vi "SCM2_T_Control_Remote.vi"() -> ()   [LabVIEW 2018]
panel:
  out "Label.Text Array":string[](array[string])
  in  "Sorb Setpoint (K)":dbl=0.3 format="%#_4g"
  in  "OK Button":bool
  in  "Data mac ip address":string="146.201.200.173"
  in  "port":u16=3376
  in  "error in (no error) 2":errorcluster
  in  "Probe Setpoint (K)":dbl=0.3 format="%#_4g"
  in  "ico":u16(ring)=1 items=["Sorb"=1, "Probe"=2, "Test"=3]
  # "ico = 1 Sorb\n       = 2 Probe"
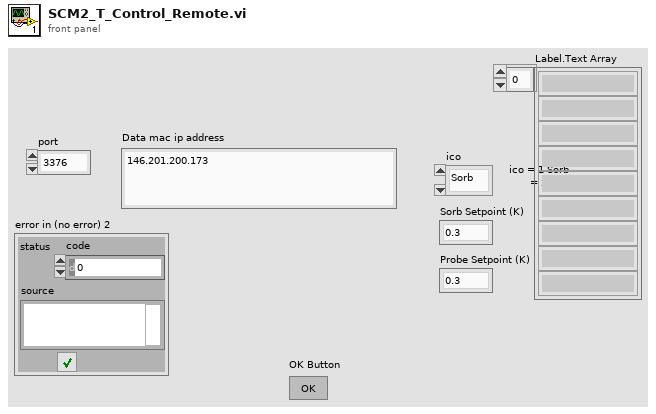
[diagram p1: front panel]
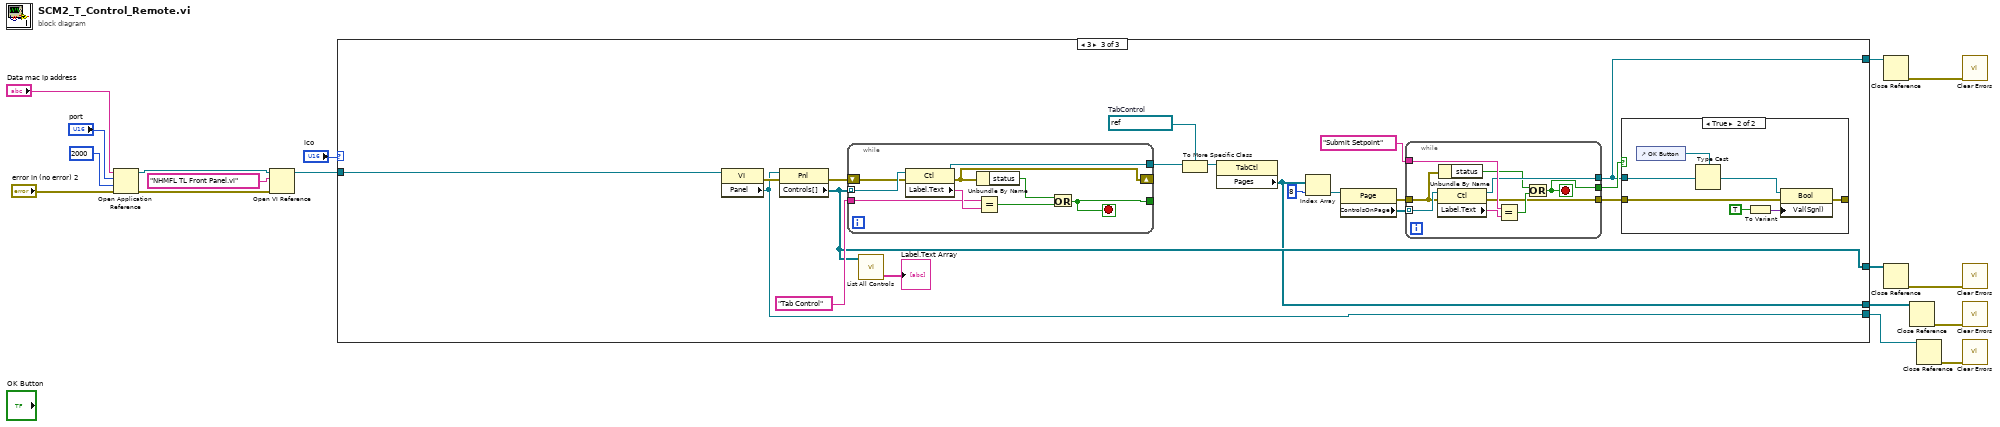
[diagram p0: block diagram]
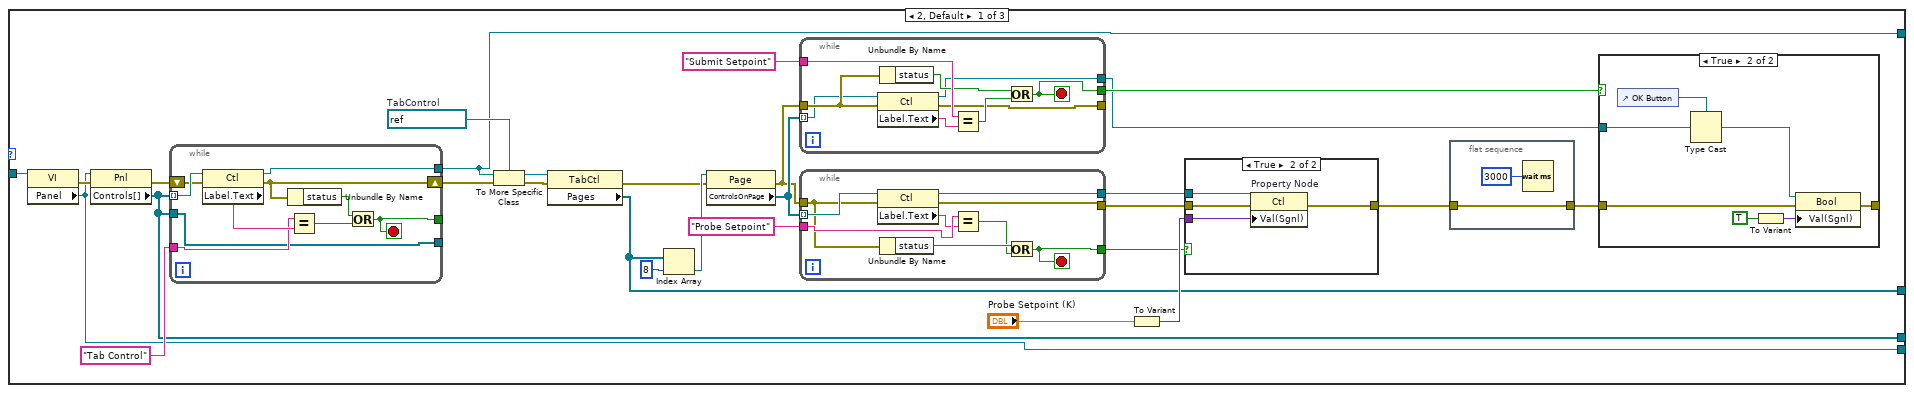
[diagram p2: hidden frame]
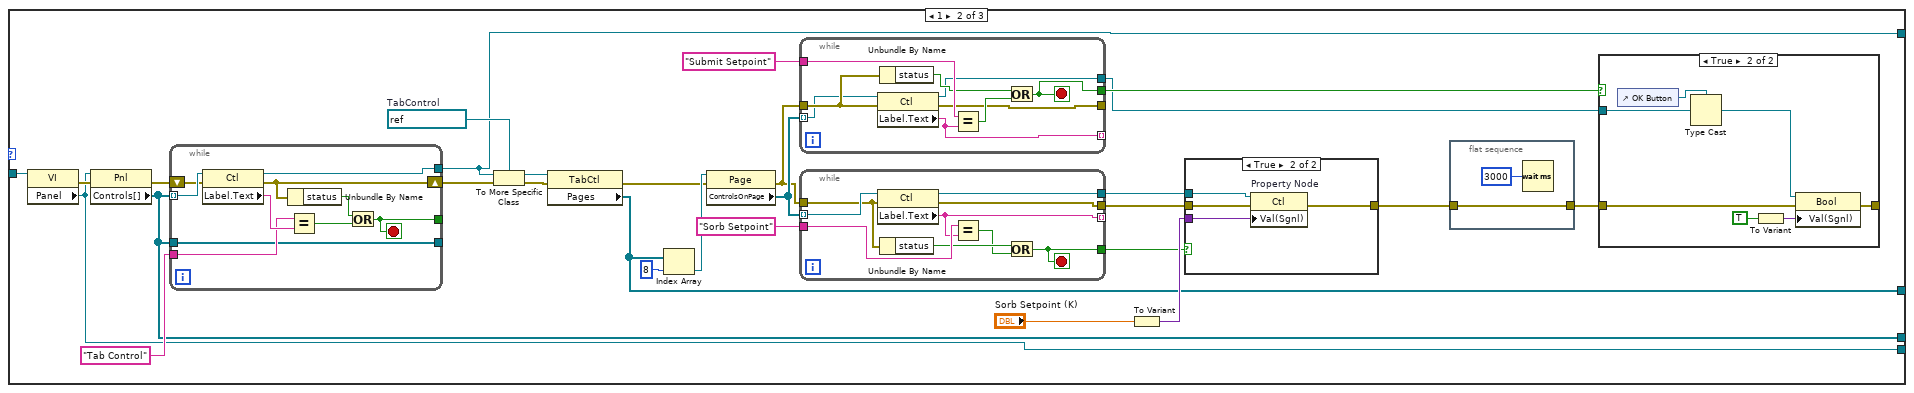
[diagram p5: hidden frame]
diagram:
  n1 = Open Application Reference(8:"error in (no error) 2", 9:2000 ("timeout ms (60000)"), 10:"port", 11:"Data mac ip address") -> (0:w4:errorcluster, 3:w5:refnum<vi>)
  n2 = Open VI Reference(application reference (local)=w5, vi path="NHMFL TL Front Panel.vi", error in (no error)=w4) -> (vi reference=w16:refnum<vi>)  [unwired: 3 in, 1 out]
  n3 = case shown="3" "ico" {
    tunnel: w16 -> [w41 w112 w177]
    tunnel: [w25 w94 w172] -> w13
    tunnel: [w26 w95 w160] -> w12
    tunnel: [w40 w111 w176] -> w11
    tunnel: [w24 w93 w161] -> w1
    frame 2, Default {
      w37 = refnum<vi> refnum  # TabControl
      n4 = property class="VI"(reference=w41) -> (error out=w45:errorcluster, "Panel"=w40:refnum<vi>)  [unwired: 1 in, 1 out]
      n5 = property class="Pnl"(reference=w40, error in=w45) -> (error out=w39:errorcluster, "Controls[]"=w26:refnum<vi>[])  [unwired: 1 out]
      n6 = while {
        tunnel: w26 -> [w88] mode=indexing
        tunnel: "Tab Control" ("Control Name") -> [w86]
        shift-right: [w83] -> w35
        shift-left: w39 -> [w85]
        tunnel: [w84] -> w25
        tunnel: [w80] -> _
        tunnel: w26 -> [w79]
        tunnel: [w79] -> _
        stop <- w80 stop-if-true
        n7 = property class="Ctl"(reference=w88, error in=w85) -> (reference out=w84:refnum<vi>, error out=w83:errorcluster, "Label.Text"=w87:string)
        n8 = Unbundle By Name(w83) -> ("status"=w82:bool)
        n9 = Equal?(x=w86, y=w87) -> (x = y?=w81:bool)
        n10 = Or(x=w82, y=w81) -> (x .or. y?=w80:bool)
      }
      n11 = To More Specific Class(target class=w37, reference=w25, error in=w35) -> (specific class reference=w38:refnum<vi>, error out=w36:errorcluster)
      n12 = property class="TabCtl"(reference=w38, error in=w36) -> (error out=w33:errorcluster, "Pages"=w24:refnum<vi>[])  [unwired: 1 out]
      n13 = Index Array(array=w24, index=8) -> (element=w34:refnum<vi>)
      n14 = property class="Page"(reference=w34, error in=w33) -> (error out=w18:errorcluster, "ControlsOnPage"=w19:refnum<vi>[])  [unwired: 1 out]
      n15 = while {
        tunnel: "Submit Setpoint" ("Control Name") -> [w56]
        tunnel: w18 -> [w51]
        tunnel: w19 -> [w49] mode=indexing
        tunnel: [w48] -> w22
        tunnel: [w53] -> w23
        tunnel: [w52] -> _
        stop <- w53 stop-if-true
        n16 = property class="Ctl"(reference=w49, error in=w51) -> (reference out=w48:refnum<vi>, error out=w52:errorcluster, "Label.Text"=w50:string)
        n17 = Unbundle By Name(w51) -> ("status"=w55:bool)
        n18 = Equal?(x=w56, y=w50) -> (x = y?=w54:bool)
        n19 = Or(x=w55, y=w54) -> (x .or. y?=w53:bool)
      }
      n20 = while {
        tunnel: "Probe Setpoint" ("Control Name") -> [w65]
        tunnel: w18 -> [w58]
        tunnel: w19 -> [w62] mode=indexing
        tunnel: [w61] -> w28
        tunnel: [w60] -> w30
        tunnel: [w59] -> w29
        stop <- w60 stop-if-true
        n21 = property class="Ctl"(reference=w62, error in=w58) -> (reference out=w61:refnum<vi>, error out=w59:errorcluster, "Label.Text"=w57:string)
        n22 = Unbundle By Name(w58) -> ("status"=w64:bool)
        n23 = Equal?(x=w65, y=w57) -> (x = y?=w63:bool)
        n24 = Or(x=w64, y=w63) -> (x .or. y?=w60:bool)
      }
      n25 = To Variant(anything="Probe Setpoint (K)") -> (Variant=w43:variant)
      n26 = case shown="True" w30 {
        tunnel: w29 -> [w74 w78]
        tunnel: [w74 w77] -> w21
        tunnel: w43 -> [_ w76]
        tunnel: w28 -> [_ w75]
        frame False {
        }
        frame True {
          n27 = property on="Property Node" class="Ctl"(reference=w75, error in=w78, "Val(Sgnl)"=w76) -> (error out=w77:errorcluster)  [unwired: 1 out]
        }
      }
      n28 = flat-sequence {
        tunnel: [w46] -> w20
        tunnel: w21 -> [w46]
        frame #0 {
          n29 = Wait (ms)(milliseconds to wait=u32 3000) -> ()  [unwired: 1 out]
        }
      }
      n30 = case shown="True" w23 {
        tunnel: w20 -> [w66 w72]
        tunnel: [w66 w71] -> _
        tunnel: w22 -> [_ w70]
        frame False {
        }
        frame True {
          n31 = control-ref of="OK Button"() -> (w73:refnum<vi>)
          n32 = Type Cast(type=w73, x=w70) -> (*(type *) &x=w69:refnum<vi>)
          n33 = To Variant(anything=TRUE) -> (Variant=w67:variant)
          n34 = property class="Bool"(reference=w69, error in=w72, "Val(Sgnl)"=w67) -> (error out=w71:errorcluster)  [unwired: 1 out]
        }
      }
    }
    frame 1 {
      w108 = refnum<vi> refnum  # TabControl
      n35 = property class="VI"(reference=w112) -> (error out=w116:errorcluster, "Panel"=w111:refnum<vi>)  [unwired: 1 in, 1 out]
      n36 = property class="Pnl"(reference=w111, error in=w116) -> (error out=w110:errorcluster, "Controls[]"=w95:refnum<vi>[])  [unwired: 1 out]
      n37 = while {
        tunnel: w95 -> [w159] mode=indexing
        tunnel: "Tab Control" ("Control Name") -> [w157]
        shift-right: [w154] -> w106
        shift-left: w110 -> [w156]
        tunnel: [w155] -> w94
        tunnel: [w151] -> _
        tunnel: w95 -> [w150]
        tunnel: [w150] -> _
        stop <- w151 stop-if-true
        n38 = property class="Ctl"(reference=w159, error in=w156) -> (reference out=w155:refnum<vi>, error out=w154:errorcluster, "Label.Text"=w158:string)
        n39 = Unbundle By Name(w154) -> ("status"=w153:bool)
        n40 = Equal?(x=w157, y=w158) -> (x = y?=w152:bool)
        n41 = Or(x=w153, y=w152) -> (x .or. y?=w151:bool)
      }
      n42 = To More Specific Class(target class=w108, reference=w94, error in=w106) -> (specific class reference=w109:refnum<vi>, error out=w107:errorcluster)
      n43 = property class="TabCtl"(reference=w109, error in=w107) -> (error out=w104:errorcluster, "Pages"=w93:refnum<vi>[])  [unwired: 1 out]
      n44 = Index Array(array=w93, index=8) -> (element=w105:refnum<vi>)
      n45 = property class="Page"(reference=w105, error in=w104) -> (error out=w97:errorcluster, "ControlsOnPage"=w98:refnum<vi>[])  [unwired: 1 out]
      n46 = while {
        tunnel: "Submit Setpoint" ("Control Name") -> [w127]
        tunnel: w97 -> [w122]
        tunnel: w98 -> [w120] mode=indexing
        tunnel: [w119] -> w91
        tunnel: [w124] -> w92
        tunnel: [w123] -> _
        tunnel: [w121] -> _ mode=indexing
        stop <- w124 stop-if-true
        n47 = property class="Ctl"(reference=w120, error in=w122) -> (reference out=w119:refnum<vi>, error out=w123:errorcluster, "Label.Text"=w121:string)
        n48 = Unbundle By Name(w122) -> ("status"=w126:bool)
        n49 = Equal?(x=w127, y=w121) -> (x = y?=w125:bool)
        n50 = Or(x=w126, y=w125) -> (x .or. y?=w124:bool)
      }
      n51 = while {
        tunnel: "Sorb Setpoint" ("Control Name") -> [w136]
        tunnel: w97 -> [w129]
        tunnel: w98 -> [w133] mode=indexing
        tunnel: [w132] -> w99
        tunnel: [w131] -> w101
        tunnel: [w130] -> w100
        tunnel: [w128] -> _ mode=indexing
        stop <- w131 stop-if-true
        n52 = property class="Ctl"(reference=w133, error in=w129) -> (reference out=w132:refnum<vi>, error out=w130:errorcluster, "Label.Text"=w128:string)
        n53 = Unbundle By Name(w129) -> ("status"=w135:bool)
        n54 = Equal?(x=w136, y=w128) -> (x = y?=w134:bool)
        n55 = Or(x=w135, y=w134) -> (x .or. y?=w131:bool)
      }
      n56 = To Variant(anything="Sorb Setpoint (K)") -> (Variant=w114:variant)
      n57 = case shown="True" w101 {
        tunnel: w100 -> [w145 w149]
        tunnel: [w145 w148] -> w90
        tunnel: w114 -> [_ w147]
        tunnel: w99 -> [_ w146]
        frame False {
        }
        frame True {
          n58 = property on="Property Node" class="Ctl"(reference=w146, error in=w149, "Val(Sgnl)"=w147) -> (error out=w148:errorcluster)  [unwired: 1 out]
        }
      }
      n59 = flat-sequence {
        tunnel: [w117] -> w89
        tunnel: w90 -> [w117]
        frame #0 {
          n60 = Wait (ms)(milliseconds to wait=u32 3000) -> ()  [unwired: 1 out]
        }
      }
      n61 = case shown="True" w92 {
        tunnel: w89 -> [w137 w143]
        tunnel: [w137 w142] -> _
        tunnel: w91 -> [_ w141]
        frame False {
        }
        frame True {
          n62 = control-ref of="OK Button"() -> (w144:refnum<vi>)
          n63 = Type Cast(type=w144, x=w141) -> (*(type *) &x=w140:refnum<vi>)
          n64 = To Variant(anything=TRUE) -> (Variant=w138:variant)
          n65 = property class="Bool"(reference=w140, error in=w143, "Val(Sgnl)"=w138) -> (error out=w142:errorcluster)  [unwired: 1 out]
        }
      }
    }
    frame 3 {
      w170 = refnum<vi> refnum  # TabControl
      n66 = property class="VI"(reference=w177) -> (error out=w178:errorcluster, "Panel"=w176:refnum<vi>)  [unwired: 1 in, 1 out]
      n67 = property class="Pnl"(reference=w176, error in=w178) -> (error out=w164:errorcluster, "Controls[]"=w161:refnum<vi>[])  [unwired: 1 out]
      n68 = while {
        tunnel: w161 -> [w187] mode=indexing
        tunnel: "Tab Control" ("Control Name") -> [w185]
        shift-right: [w182] -> _
        shift-left: w164 -> [w184]
        tunnel: [w183] -> w166
        tunnel: [w179] -> _
        stop <- w179 stop-if-true
        n69 = property class="Ctl"(reference=w187, error in=w184) -> (reference out=w183:refnum<vi>, error out=w182:errorcluster, "Label.Text"=w186:string)
        n70 = Unbundle By Name(w182) -> ("status"=w181:bool)
        n71 = Equal?(x=w185, y=w186) -> (x = y?=w180:bool)
        n72 = Or(x=w181, y=w180) -> (x .or. y?=w179:bool)
      }
      n73 = call "List All Controls.vi"("Ref Controls[]"=w161) -> ("Label.Text Array"=→"Label.Text Array":string[])  [unwired: 3 in, 1 out]
      n74 = To More Specific Class(target class=w170, reference=w166) -> (specific class reference=w165:refnum<vi>)  [unwired: 1 in, 1 out]
      n75 = property class="TabCtl"(reference=w165) -> ("Pages"=w160:refnum<vi>[])  [unwired: 1 in, 2 out]
      n76 = Index Array(array=w160, index=8) -> (element=w168:refnum<vi>)
      n77 = property class="Page"(reference=w168) -> (error out=w162:errorcluster, "ControlsOnPage"=w163:refnum<vi>[])  [unwired: 1 in, 1 out]
      n78 = while {
        tunnel: "Submit Setpoint" ("Control Name") -> [w196]
        tunnel: [w191] -> w172
        tunnel: [w194] -> w174
        tunnel: [w193] -> w173
        tunnel: w162 -> [w188]
        tunnel: w163 -> [w190] mode=indexing
        stop <- w194 stop-if-true
        n79 = property class="Ctl"(reference=w190, error in=w188) -> (reference out=w191:refnum<vi>, error out=w193:errorcluster, "Label.Text"=w192:string)
        n80 = Unbundle By Name(w188) -> ("status"=w189:bool)
        n81 = Equal?(x=w196, y=w192) -> (x = y?=w195:bool)
        n82 = Or(x=w189, y=w195) -> (x .or. y?=w194:bool)
      }
      n83 = case shown="True" w174 {
        tunnel: w173 -> [w197 w203]
        tunnel: [w197 w202] -> _
        tunnel: w172 -> [_ w198]
        frame False {
        }
        frame True {
          n84 = control-ref of="OK Button"() -> (w204:refnum<vi>)
          n85 = Type Cast(type=w204, x=w198) -> (*(type *) &x=w201:refnum<vi>)
          n86 = To Variant(anything=TRUE) -> (Variant=w199:variant)
          n87 = property class="Bool"(reference=w201, error in=w203, "Val(Sgnl)"=w199) -> (error out=w202:errorcluster)  [unwired: 1 out]
        }
      }
    }
  }
  n88 = Close Reference(reference=w13) -> (error out=w17:errorcluster)  [unwired: 1 in]
  n89 = Close Reference(reference=w1) -> (error out=w2:errorcluster)  [unwired: 1 in]
  n90 = Close Reference(reference=w12) -> (error out=w15:errorcluster)  [unwired: 1 in]
  n91 = Close Reference(reference=w11) -> (error out=w14:errorcluster)  [unwired: 1 in]
  n92 = call <vilib>:"Clear Errors.vi"("error in (no error)"=w17) -> ()  [unwired: 5 in, 2 out]
  n93 = call <vilib>:"Clear Errors.vi"("error in (no error)"=w2) -> ()  [unwired: 5 in, 2 out]
  n94 = call <vilib>:"Clear Errors.vi"("error in (no error)"=w15) -> ()  [unwired: 5 in, 2 out]
  n95 = call <vilib>:"Clear Errors.vi"("error in (no error)"=w14) -> ()  [unwired: 5 in, 2 out]
